vi "PopulateSingleFrame.vi"(6 "New Image Size\nwhen != 0":T1={"X Size"=0, "Y Size"=0, "adc_res"=0, "NoOfRoutingChannel"=1}, 8 "Error In":errorcluster, 10 "EventData":u16[](array[numeric]) format="%04x") -> (0 "Error Out":errorcluster, 2 "DecaySum":u32[](array[numeric]), 3 "CounterCluster":T2={"Pixel No"=0, "Frame No"=-1, "LastPixelTime"=0, "Line No"=-1, "StopFrame"=FALSE, "StartFrame"=FALSE, "Frame Flag"=FALSE, "Out Of Y"=FALSE, "MT-Overflow"=FALSE, "Photon Count"=0, "LineLength"=0, "FrameHeight"=0, "MT-Overflow"=0, "PixelDwellTime"=0}, 4 "DecayMatrix":u16[][][][](array[numeric]), 5 "IntensityGraph":u32[][](graph))   [LabVIEW 2019]
doc: "This VI goes through an EventData-Array received from 'SPC_read_fifo.vi' and interprets the events as markers or photons and populates a DecayMatrix for a single frame.\nThe 4 dimensions of DecayMatrix are the decay curves according to the microTime values of photons, in their image X- and Y-axis position and routing channel.\nNote the two possible ways of creating an IntensityGraph: With every photon event the intensity could increase per X-Y-coordinate, or the really counted photon number during a pixel event is used (usually higher).\nA functional global variable concept is used to initialize the control cluster and output arrays.\nThis VI accumulates only events for one frame.\nA similar VI used at the executable example 'ImagingEventStream-FifoImage.exe' that also collects multiple frames with improved memory management is available at B&H.\n\ninfo@becker-hickl.com"
uses:
  SPC_Controls/Fifo_CounterCluster.ctl
panel:
  out "BufferedImageSize":T1={"X Size"=0, "Y Size"=0, "adc_res"=0, "NoOfRoutingChannel"=1}
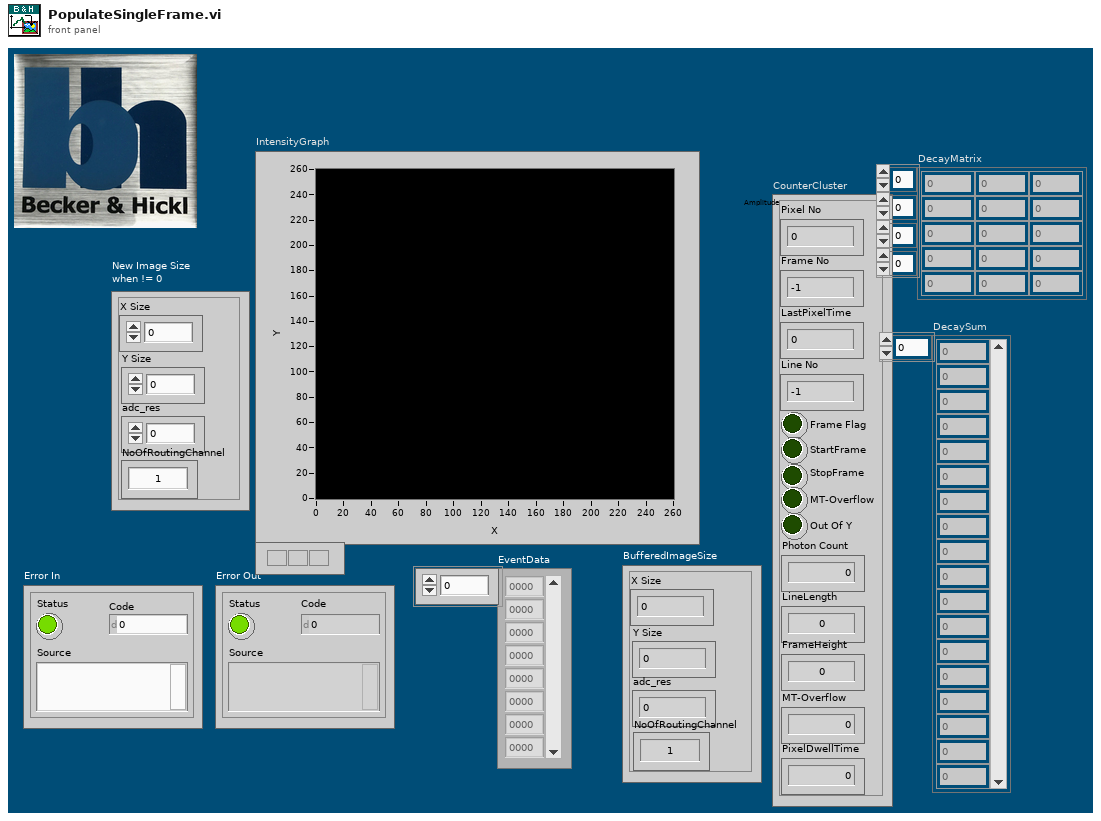
[diagram p1: front panel]
types:
  T1 = cluster{"X Size":i32, "Y Size":i32, "adc_res":i32, "NoOfRoutingChannel":i32}
  T2 = typedef "Fifo_CounterCluster.ctl" = cluster{"Pixel No":i32, "Frame No":i32, "LastPixelTime":i32, "Line No":i32, "StopFrame":bool, "StartFrame":bool, "Frame Flag":bool, "Out Of Y":bool, "MT-Overflow":bool, "Photon Count":u64, "LineLength":i32, "FrameHeight":i32, "MT-Overflow":u32, "PixelDwellTime":u32}
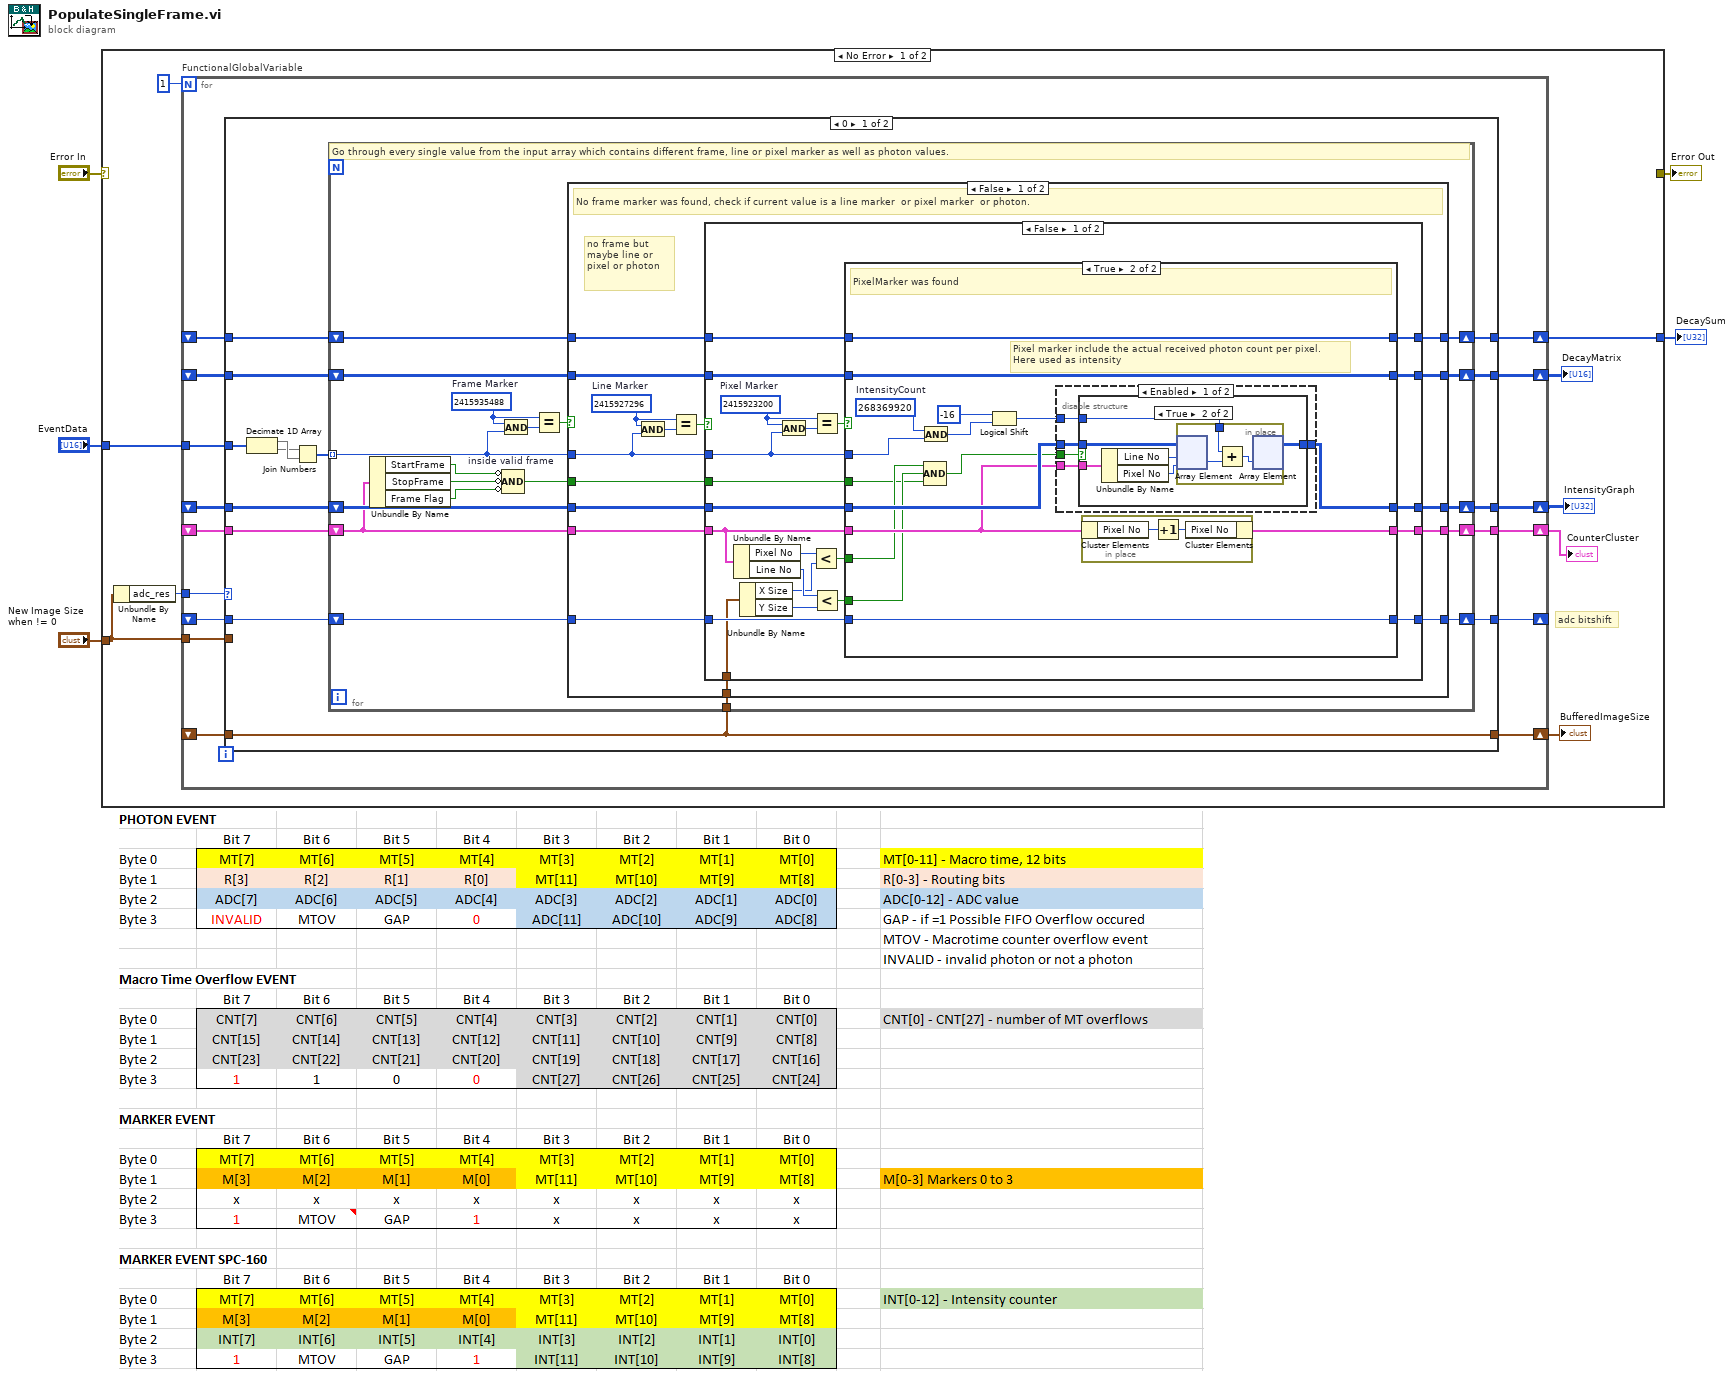
[diagram p0: block diagram]
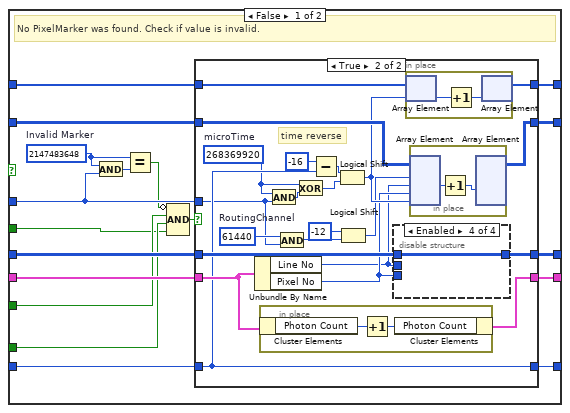
[diagram p2: hidden frame]
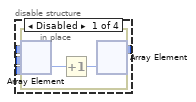
[diagram p4: hidden frame]
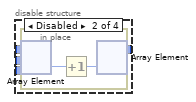
[diagram p5: hidden frame]
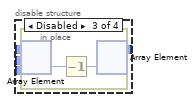
[diagram p6: hidden frame]
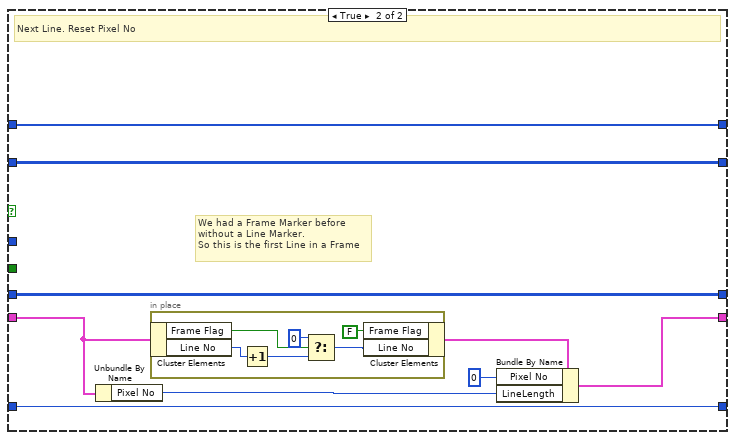
[diagram p9: hidden frame]
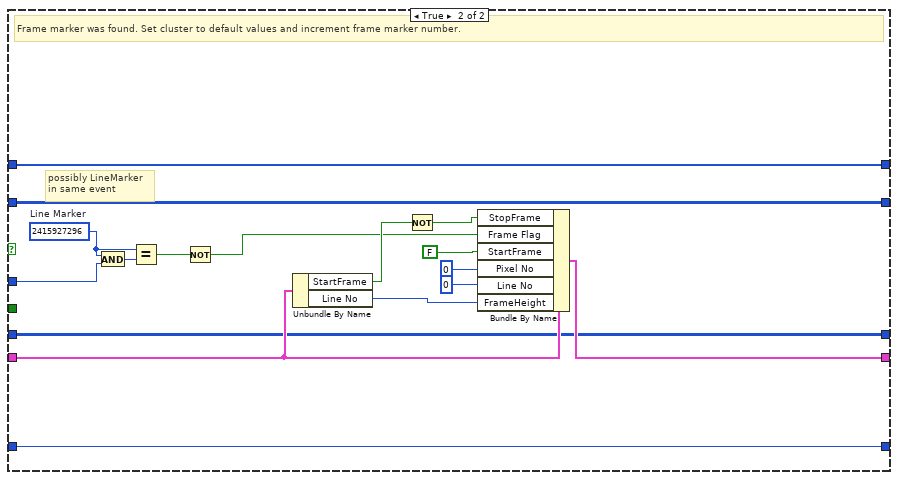
[diagram p10: hidden frame]
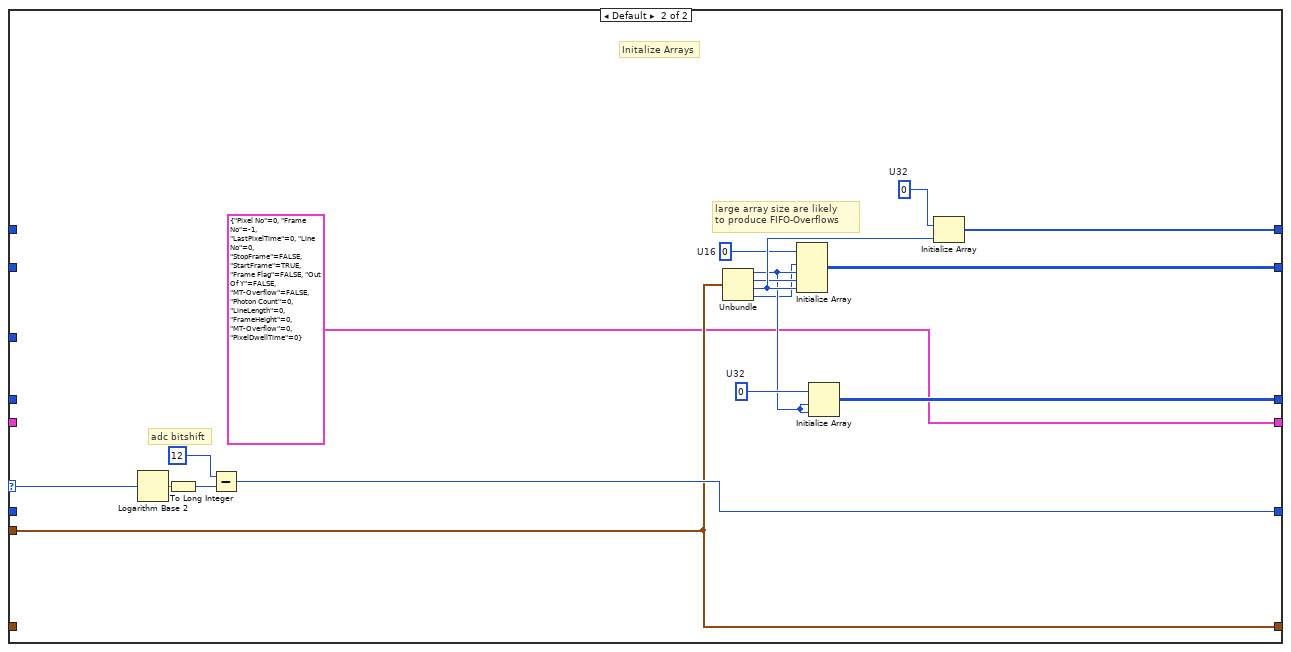
[diagram p11: hidden frame]
diagram:
  n1 = case shown="No Error" "Error In" {
    selector: "Error In" -> [_ w255]
    tunnel: [_ w255] -> w4
    tunnel: "New Image Size\nwhen != 0" -> [w11 _]
    tunnel: "EventData" -> [w14 _]
    tunnel: [w10 _] -> w1
    frame No Error {
      # "adc bitshift"
      n2 = Unbundle By Name(w11) -> ("adc_res"=w13:i32)
      n3 = for "FunctionalGlobalVariable" {
        N: 1 -> [_]
        tunnel: w14 -> [w25]
        shift-right: [w29] -> w8
        shift-left: _ -> [w24]
        tunnel: w13 -> [w21]
        shift-right: [w20] -> w9
        shift-left: _ -> [w26]
        tunnel: w11 -> [w19]
        shift-right: [w27] -> w6
        shift-left: _ -> [w28]
        shift-right: [w18] -> w10
        shift-left: _ -> [w17]
        shift-right: [w16] -> _
        shift-left: _ -> [w15]
        shift-right: [w22] -> w7
        shift-left: _ -> [w23]
        n4 = case shown="0" w21 {
          selector: w21 -> [_ w246]
          tunnel: [w43 T2 {"Pixel No"=0, "Frame No"=-1, "LastPixelTime"=0, "Line No"=0, "StopFrame"=FALSE, "StartFrame"=TRUE, "Frame Flag"=FALSE, "Out Of Y"=FALSE, "MT-Overflow"=FALSE, "Photon Count"=0, "LineLength"=0, "FrameHeight"=0, "MT-Overflow"=0, "PixelDwellTime"=0} ("Counter Cluster")] -> w29
          tunnel: w28 -> [w42 _]
          tunnel: [w41 w254] -> w27
          tunnel: w26 -> [w31 _]
          tunnel: w25 -> [w40 _]
          tunnel: w24 -> [w30 _]
          tunnel: w23 -> [w37 _]
          tunnel: [w36 w243] -> w22
          tunnel: [w31 w239] -> w20
          tunnel: w19 -> [_ w239]
          tunnel: [w34 w251] -> w18
          tunnel: w17 -> [w35 _]
          tunnel: [w32 w245] -> w16
          tunnel: w15 -> [w33 _]
          frame 0 {
            n5 = Decimate 1D Array(w40) -> (w39:u16[], w38:u16[])
            n6 = Join Numbers(hi=w38, lo=w39) -> ((hi.lo)=w44:u32[])
            n7 = for {
              tunnel: w44 -> [w50] mode=indexing
              shift-right: [w60] -> w43
              shift-left: w30 -> [w45]
              shift-right: [w58] -> w36
              shift-left: w37 -> [w59]
              shift-right: [w57] -> w41
              shift-left: w42 -> [w56]
              tunnel: w31 -> [w55]
              shift-right: [w53] -> w34
              shift-left: w35 -> [w54]
              shift-right: [w51] -> w32
              shift-left: w33 -> [w52]
              w63 = u32 2415935488  # Frame Marker
              # "Go through every single value from the input array which contains different frame, line or pixel marker as well as photon values."
              n8 = Unbundle By Name(w45) -> ("StartFrame"=w49:bool, "StopFrame"=w48:bool, "Frame Flag"=w47:bool)
              n9 = And(x=w63, y=w50) -> (x .and. y?=w62:u32)
              n10 = Compound Arithmetic op=AND "inside valid frame"(invert w49, invert w48, invert w47) -> (w46:bool)
              n11 = Equal?(x=w63, y=w62) -> (x = y?=w61:bool)
              n12 = case shown="False" w61 {
                tunnel: w45 -> [w77 w234]
                tunnel: [w76 w237] -> w60
                tunnel: w50 -> [w71 w230]
                tunnel: w59 -> [w75 w223]
                tunnel: [w74 w223] -> w58
                tunnel: [w73 w233] -> w57
                tunnel: w56 -> [w72 w233]
                tunnel: w55 -> [w69 _]
                tunnel: w54 -> [w68 w228]
                tunnel: [w67 w228] -> w53
                tunnel: w52 -> [w66 w227]
                tunnel: [w65 w227] -> w51
                tunnel: w46 -> [w64 _]
                frame False {
                  w78 = u32 2415927296  # Line Marker
                  # "no frame but maybe line or pixel or photon"
                  # "No frame marker was found, check if current value is a line marker  or pixel marker  or photon."
                  n13 = And(x=w78, y=w71) -> (x .and. y?=w79:u32)
                  n14 = Equal?(x=w78, y=w79) -> (x = y?=w70:bool)
                  n15 = case shown="False" w70 {
                    tunnel: w77 -> [w81 w210]
                    tunnel: [w99 w213] -> w76
                    tunnel: w71 -> [w95 _]
                    tunnel: w75 -> [w98 w212]
                    tunnel: [w97 w212] -> w74
                    tunnel: [w94 w211] -> w73
                    tunnel: w72 -> [w93 w211]
                    tunnel: w69 -> [w84 _]
                    tunnel: w68 -> [w92 w207]
                    tunnel: [w91 w207] -> w67
                    tunnel: w66 -> [w85 w206]
                    tunnel: [w90 w206] -> w65
                    tunnel: w64 -> [w80 _]
                    frame False {
                      w100 = u32 2415923200  # Pixel Marker
                      n16 = Unbundle By Name(w81) -> ("Pixel No"=w86:i32, "Line No"=w89:i32)
                      n17 = Unbundle By Name(w84) -> ("X Size"=w87:i32, "Y Size"=w88:i32)
                      n18 = And(x=w100, y=w95) -> (x .and. y?=w101:u32)
                      n19 = Less?(x=w86, y=w87) -> (x < y?=w82:bool)
                      n20 = Equal?(x=w100, y=w101) -> (x = y?=w96:bool)
                      n21 = Less?(x=w89, y=w88) -> (x < y?=w83:bool)
                      n22 = case shown="True" w96 {
                        tunnel: [w115 w186] -> w99
                        tunnel: w81 -> [w111 w181]
                        tunnel: w98 -> [w119 w183]
                        tunnel: [w118 w182] -> w97
                        tunnel: w95 -> [w107 w179]
                        tunnel: [w116 w187] -> w94
                        tunnel: w93 -> [w117 w187]
                        tunnel: w92 -> [w114 w185]
                        tunnel: [w113 w185] -> w91
                        tunnel: w85 -> [w110 w184]
                        tunnel: [w112 w184] -> w90
                        tunnel: w83 -> [w109 w174]
                        tunnel: w82 -> [w108 w175]
                        tunnel: w80 -> [w102 w172]
                        frame False {
                          w106 = u32 2147483648  # Invalid Marker
                          # "No PixelMarker was found. Check if value is invalid."
                          n23 = And(x=w106, y=w107) -> (x .and. y?=w105:u32)
                          n24 = Equal?(x=w106, y=w105) -> (x = y?=w104:bool)
                          n25 = Compound Arithmetic op=AND(invert w104, w108, w109, w102) -> (w103:bool)
                          n26 = case shown="True" w103 {
                            tunnel: w119 -> [w124 w146]
                            tunnel: [w124 w145] -> w118
                            tunnel: w111 -> [w122 w140]
                            tunnel: w117 -> [w123 w144]
                            tunnel: [w123 w143] -> w116
                            tunnel: w107 -> [_ w131]
                            tunnel: [w122 w139] -> w115
                            tunnel: w114 -> [w121 w135]
                            tunnel: [w121 w138] -> w113
                            tunnel: w110 -> [w120 w136]
                            tunnel: [w120 w136] -> w112
                            frame False {
                            }
                            frame True {
                              w132 = u32 61440  # RoutingChannel
                              w133 = u32 268369920  # microTime
                              # "time reverse"
                              n27 = Unbundle By Name(w140) -> ("Line No"=w126:i32, "Pixel No"=w127:i32)
                              n28 = in-place {
                                n29 = in-place-cluster #1(w140) -> ("Photon Count"=w171:u64)
                                n30 = Increment(x=w171) -> (x+1=w170:u64)
                                n31 = in-place-cluster #1("Photon Count"=w170) -> (w139:T2)
                              }
                              n32 = And(x=w133, y=w131) -> (x .and. y?=w141:u32)
                              n33 = And(x=w132, y=w131) -> (x .and. y?=w130:u32)
                              n34 = Exclusive Or(1:w141, 2:w133) -> (0:w134:u32)
                              n35 = Subtract(x=-16, y=w136) -> (x-y=w137:i32)
                              n36 = Logical Shift(y=w137, x=w134) -> (x << y=w128:u32)
                              n37 = Logical Shift(y=i16 -12, x=w130) -> (x << y=w125:u32)
                              n38 = disable-structure shown="Enabled" {
                                disable-tunnel: w146 -> [w152 w158 w164 w167]
                                disable-tunnel: [w151 w157 w163 w167] -> w145
                                disable-tunnel: w126 -> [w150 w156 w162 _]
                                disable-tunnel: w127 -> [w149 w155 w161 _]
                                frame Disabled {
                                n39 = in-place {
                                n40 = in-place-array #2(w152, w150, w149) -> (w154:u32)
                                n41 = Increment(x=w154) -> (x+1=w153:u32)
                                n42 = in-place-array #2(w153) -> (w151:u32[][])  [unwired: 2 out]
                                }
                                }
                                frame Disabled {
                                n43 = in-place {
                                n44 = in-place-array #3(w158, w156, w155) -> (w160:u32)
                                n45 = Increment(x=w160) -> (x+1=w159:u32)
                                n46 = in-place-array #3(w159) -> (w157:u32[][])  [unwired: 2 out]
                                }
                                }
                                frame Disabled {
                                n47 = in-place {
                                n48 = in-place-array #4(w164, w162, w161) -> (w166:u32)
                                n49 = Decrement(x=w166) -> (x-1=w165:u32)
                                n50 = in-place-array #4(w165) -> (w163:u32[][])  [unwired: 2 out]
                                }
                                }
                                frame Enabled {
                                }
                              }
                              n51 = in-place {
                                n52 = in-place-array #5(w135, w128) -> (w169:u32)
                                n53 = Increment(x=w169) -> (x+1=w168:u32)
                                n54 = in-place-array #5(w168) -> (w138:u32[])  [unwired: 1 out]
                              }
                              n55 = in-place {
                                n56 = in-place-array #6(w144, w125, w126, w127, w128) -> (w148:u16)
                                n57 = Increment(x=w148) -> (x+1=w147:u16)
                                n58 = in-place-array #6(w147) -> (w143:u16[][][][])  [unwired: 4 out]
                              }
                            }
                          }
                        }
                        frame True {
                          w180 = u32 268369920  # IntensityCount
                          # "Pixel marker include the actual received photon count per pixel.\nHere used as intensity"
                          # "PixelMarker was found"
                          n59 = And(x=w180, y=w179) -> (x .and. y?=w177:u32)
                          n60 = Compound Arithmetic op=AND(w175, w174, w172) -> (w173:bool)
                          n61 = Logical Shift(y=-16, x=w177) -> (x << y=w176:u32)
                          n62 = disable-structure shown="Enabled" {
                            disable-tunnel: w183 -> [w192 w203]
                            disable-tunnel: [w191 w203] -> w182
                            disable-tunnel: w181 -> [w190 _]
                            disable-tunnel: w176 -> [w189 _]
                            disable-tunnel: w173 -> [w188 _]
                            frame Enabled {
                              n63 = case shown="True" w188 {
                                tunnel: w192 -> [w193 w199]
                                tunnel: [w193 w198] -> w191
                                tunnel: w190 -> [_ w197]
                                tunnel: w189 -> [_ w196]
                                frame False {
                                }
                                frame True {
                                n64 = Unbundle By Name(w197) -> ("Line No"=w195:i32, "Pixel No"=w194:i32)
                                n65 = in-place {
                                in-place-border: w196 -> [w200]
                                n66 = in-place-array #7(w199, w195, w194) -> (w202:u32)
                                n67 = Add(x=w200, y=w202) -> (x+y=w201:u32)
                                n68 = in-place-array #7(w201) -> (w198:u32[][])  [unwired: 2 out]
                                }
                                }
                              }
                            }
                            frame Disabled {
                            }
                          }
                          n69 = in-place {
                            n70 = in-place-cluster #8(w181) -> ("Pixel No"=w205:i32)
                            n71 = Increment(x=w205) -> (x+1=w204:i32)
                            n72 = in-place-cluster #8("Pixel No"=w204) -> (w186:T2)
                          }
                        }
                      }
                    }
                    frame True {
                      # "We had a Frame Marker before\nwithout a Line Marker.\nSo this is the first Line in a Frame"
                      # "Next Line. Reset Pixel No"
                      n73 = Unbundle By Name(w210) -> ("Pixel No"=w208:i32)
                      n74 = in-place {
                        n75 = in-place-cluster #9(w210) -> ("Frame Flag"=w219:bool, "Line No"=w216:i32)
                        n76 = Increment(x=w216) -> (x+1=w215:i32)
                        n77 = Select(t=0, s=w219, f=w215) -> (s? t:f=w220:i32)
                        n78 = in-place-cluster #9("Frame Flag"=FALSE, "Line No"=w220) -> (w209:T2)
                      }
                      n79 = Bundle By Name(cluster=w209, "Pixel No"=0, "LineLength"=w208) -> (w213:T2)
                    }
                  }
                }
                frame True {
                  w231 = u32 2415927296  # Line Marker
                  # "possibly LineMarker\nin same event"
                  # "Frame marker was found. Set cluster to default values and increment frame marker number."
                  n80 = And(x=w231, y=w230) -> (x .and. y?=w232:u32)
                  n81 = Equal?(x=w231, y=w232) -> (x = y?=w226:bool)
                  n82 = Not(x=w226) -> (.not. x?=w221:bool)
                  n83 = Unbundle By Name(w234) -> ("StartFrame"=w225:bool, "Line No"=w229:i32)
                  n84 = Not(x=w225) -> (.not. x?=w222:bool)
                  n85 = Bundle By Name(cluster=w234, "StopFrame"=w222, "Frame Flag"=w221, "StartFrame"=FALSE, "Pixel No"=0, "Line No"=0, "FrameHeight"=w229) -> (w237:T2)
                }
              }
            }
          }
          frame Default {
            w241 = u16 0  # U16
            w244 = u32 0  # U32
            w253 = u32 0  # U32
            # "large array size are likely\nto produce FIFO-Overflows"
            # "adc bitshift"
            # "Initalize Arrays"
            n86 = Logarithm Base 2(1:w246) -> (0:w247:dbl)
            n87 = To Long Integer(number=w247) -> (32bit integer=w248:i32)
            n88 = Subtract(x=12, y=w248) -> (x-y=w245:i32)
            n89 = Unbundle(w239) -> ("X Size"=w242:i32, "Y Size"=w250:i32, "adc_res"=w252:i32, "NoOfRoutingChannel"=w240:i32)
            n90 = Initialize Array(w241, w240, w242, w250, w252) -> (w254:u16[][][][])
            n91 = Initialize Array(w244, w242, w242) -> (w243:u32[][])
            n92 = Initialize Array(w253, w252) -> (w251:u32[])
          }
        }
      }
      "CounterCluster" <- w8
      "BufferedImageSize" <- w9
      "IntensityGraph" <- w7
      "DecayMatrix" <- w6
    }
    frame Error {
    }
  }
  "Error Out" <- w4
  "DecaySum" <- w1
